vi "errorHandlerTCP.vi"(7 "show popup":bool, 8 "error in":errorcluster, 9 "language":i32, 10 "error number":i32, 11 "connection ID":refnum<k5>) -> (0 "error out":errorcluster, 3 "connection ID":refnum<k5>)   [LabVIEW 2016]
panel:
  out "params_cluster":cluster{"language":i32, "errNbr":i32}
  in  "Params_cluster":cluster{"integer":i32, "integer":i32}
  in  "results_cluster":cluster{"errNo":i32, "string":string}
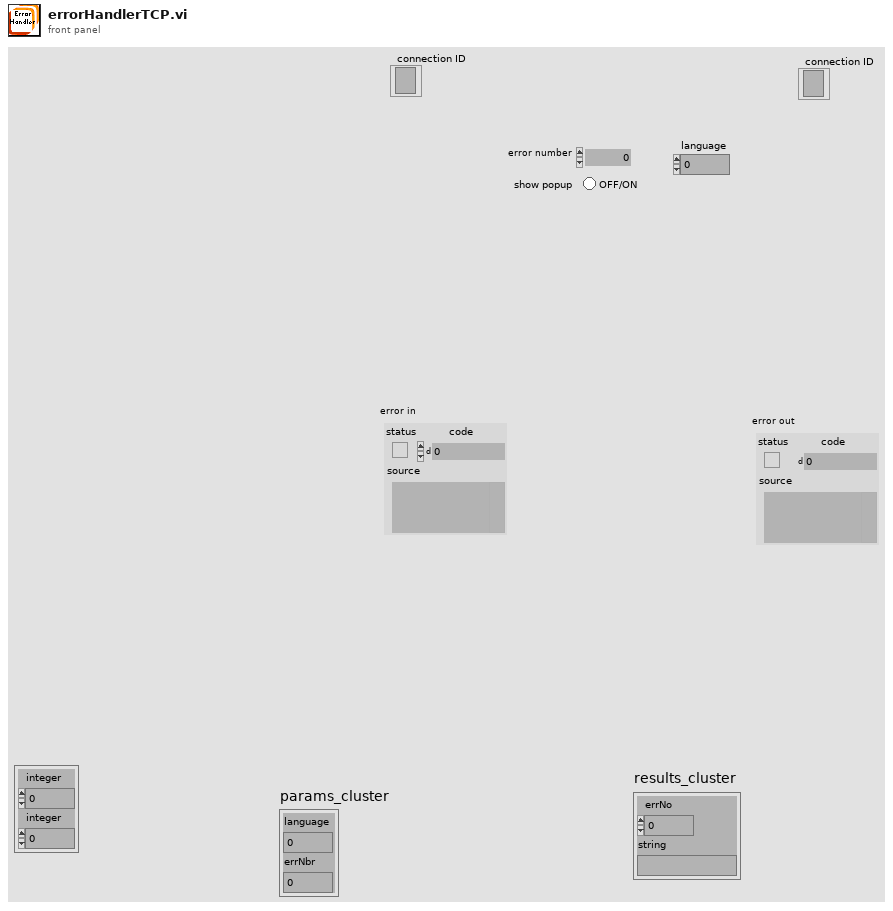
[diagram p1: front panel]
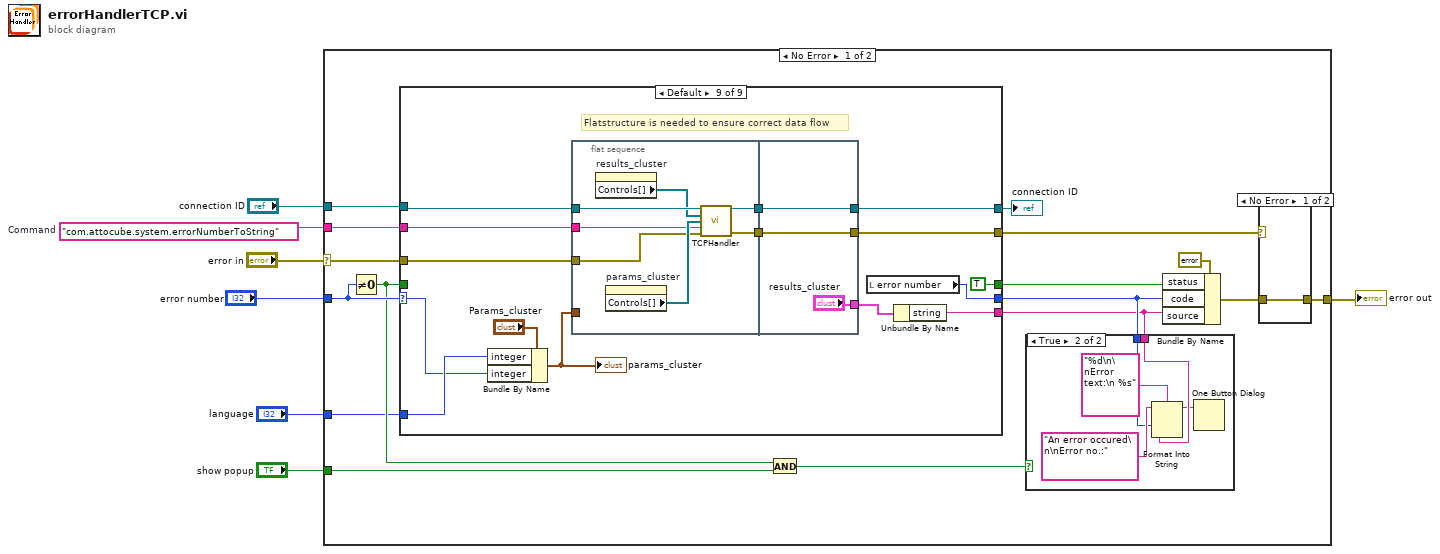
[diagram p0: block diagram]
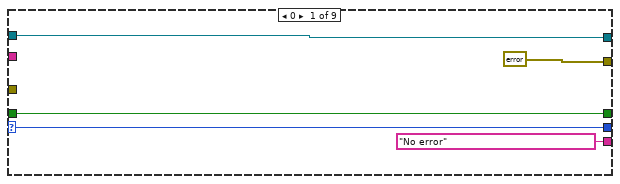
[diagram p4: hidden frame]
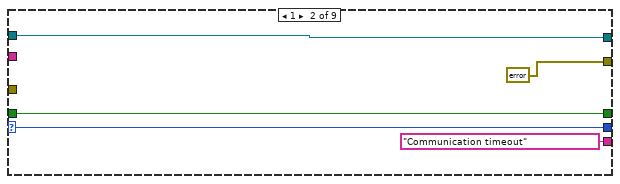
[diagram p5: hidden frame]
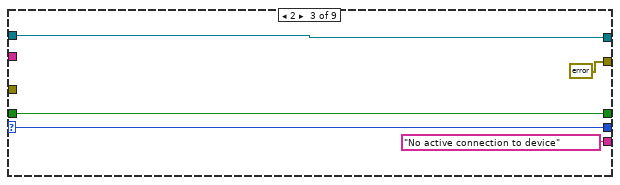
[diagram p6: hidden frame]
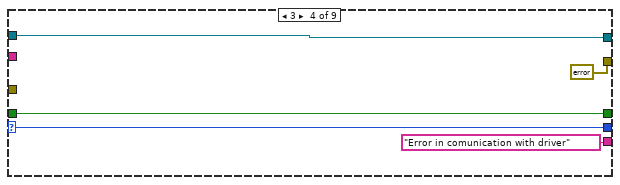
[diagram p7: hidden frame]
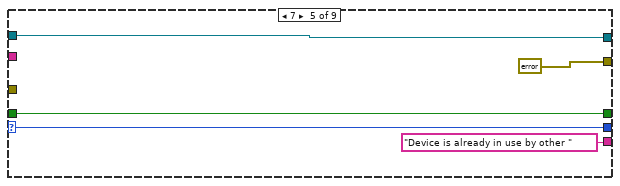
[diagram p8: hidden frame]
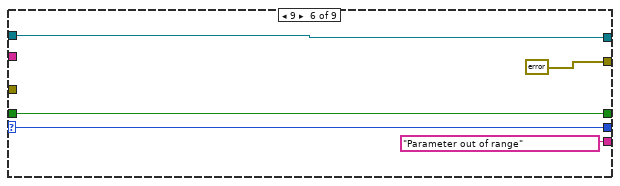
[diagram p9: hidden frame]
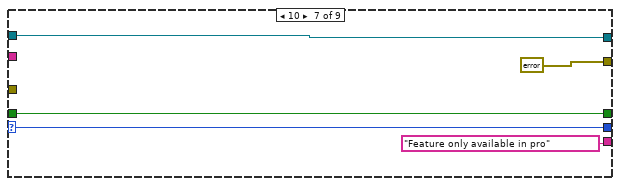
[diagram p10: hidden frame]
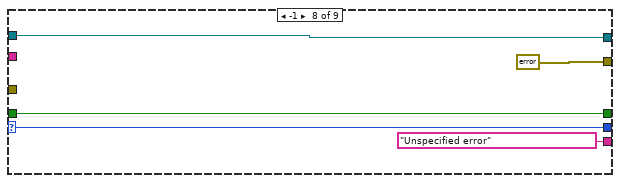
[diagram p11: hidden frame]
diagram:
  w1 = "com.attocube.system.errorNumberToString"  # Command
  n1 = case shown="No Error" "error in" {
    selector: "error in" -> [w9 w96]
    tunnel: "error number" -> [w23 _]
    tunnel: "show popup" -> [w18 _]
    tunnel: "language" -> [w16 _]
    tunnel: [w10 w96] -> w4
    tunnel: "connection ID" -> [w13 _]
    tunnel: w1 -> [w8 _]
    frame No Error {
      n2 = Not Equal To 0?(x=w23) -> (x != 0?=w19:bool)
      n3 = case shown="Default" w23 {
        selector: w23 -> [w34 w40 w44 w49 w54 w59 w64 w69 w78]
        tunnel: ["No error" "Communication timeout" "No active connection to device" "Error in comunication with driver" "Device is already in use by other " "Parameter out of range" "Feature only available in pro" "Unspecified error" w72] -> w20
        tunnel: [w34 w40 w44 w49 w54 w59 w64 w69 w71] -> w21
        tunnel: [w33 w39 w43 w50 w55 w60 w63 w70 TRUE] -> w22
        tunnel: w19 -> [w33 w39 w43 w50 w55 w60 w63 w70 _]
        tunnel: w16 -> [_ _ _ _ _ _ _ _ w79]
        tunnel: w13 -> [w32 w37 w42 w47 w52 w57 w62 w67 w77]
        tunnel: [w32 w37 w42 w47 w52 w57 w62 w67 w76] -> w15
        tunnel: [errorcluster {"status"=FALSE, "code"=0, "source"=""} ("error in") errorcluster {"status"=FALSE, "code"=0, "source"=""} ("error in") errorcluster {"status"=FALSE, "code"=0, "source"=""} ("error in") errorcluster {"status"=FALSE, "code"=0, "source"=""} ("error in") errorcluster {"status"=FALSE, "code"=0, "source"=""} ("error in") errorcluster {"status"=FALSE, "code"=0, "source"=""} ("error in") errorcluster {"status"=FALSE, "code"=0, "source"=""} ("error in") errorcluster {"status"=FALSE, "code"=0, "source"=""} ("error in") w75] -> w12
        tunnel: w9 -> [_ _ _ _ _ _ _ _ w74]
        tunnel: w8 -> [_ _ _ _ _ _ _ _ w73]
        frame 0 {
        }
        frame 1 {
        }
        frame 2 {
        }
        frame 3 {
        }
        frame 7 {
        }
        frame 9 {
        }
        frame 10 {
        }
        frame -1 {
        }
        frame Default {
          # "Flatstructure is needed to ensure correct data flow"
          n4 = Bundle By Name(cluster="Params_cluster", "integer"=w79, "integer"=w78) -> (w80:cluster{"integer":i32, "integer":i32})
          "params_cluster" <- w80
          n5 = flat-sequence {
            tunnel: [w91] -> w84
            tunnel: w77 -> [w92]
            tunnel: w73 -> [w88]
            tunnel: [w87] -> w83
            tunnel: w80 -> [_]
            tunnel: w74 -> [w86]
            tunnel: ["results_cluster"] -> w82
            tunnel: [w95] -> w76
            tunnel: w84 -> [w95]
            tunnel: [w93] -> w75
            tunnel: w83 -> [w93]
            frame #0 {
              n6 = property on="results_cluster" class="Clust (strict)"() -> ("Controls[]"=w90:refnum<vi>[])  [unwired: 2 in, 2 out]
              n7 = property on="params_cluster" class="Clust (strict)"() -> ("Controls[]"=w89:refnum<vi>[])  [unwired: 2 in, 2 out]
              n8 = call "TCPHandler.vi"("connection ID"=w92, "results_cluster"=w90, "params_cluster"=w89, "method"=w88, "error"=w86) -> ("connection ID"=w91:refnum<k5>, "error"=w87:errorcluster)  [unwired: 7 in, 2 out]
            }
            frame #1 {
            }
          }
          n9 = local read "error number"() -> (w71:i32)
          n10 = Unbundle By Name(w82) -> ("string"=w72:string)
        }
      }
      "connection ID" <- w15
      n11 = And(x=w19, y=w18) -> (x .and. y?=w17:bool)
      n12 = case shown="True" w17 {
        tunnel: w21 -> [_ w29]
        tunnel: w20 -> [_ w27]
        frame False {
        }
        frame True {
          n13 = Format Into String(format string="%d\n\nError text:\n %s", initial string="An error occured\n\nError no.:", w29, w27) -> (resulting string=w26:string)  [unwired: 1 in, 1 out]
          n14 = One Button Dialog(message=w26) -> ()  [unwired: 1 in, 1 out]
        }
      }
      n15 = Bundle By Name(cluster=errorcluster {"status"=FALSE, "code"=0, "source"=""} ("error in"), "status"=w22, "code"=w21, "source"=w20) -> (w11:errorcluster)
      n16 = case shown="No Error" w12 {
        selector: w12 -> [_ w25]
        tunnel: w11 -> [w24 _]
        tunnel: [w24 w25] -> w10
        frame No Error {
        }
        frame Error {
        }
      }
    }
    frame Error {
    }
  }
  "error out" <- w4
